vi "Parse Response Message.vi"(8 "error in":errorcluster, 11 "Luminos in":refnum<class "Luminos.lvclass">) -> (0 "error out":errorcluster, 3 "Luminos out":refnum<class "Luminos.lvclass">)   [LabVIEW 2018, in "Luminos.lvlib" / "Luminos.lvclass"]
uses:
  Luminos.lvclass
  Luminos.lvclass/Luminos.ctl
  PPLs/Axis/Axis.lvlibp/Axis.lvclass
  C:/Projects/LabVIEW/PPLs/Axis/Axis.lvlibp/Axis.lvclass
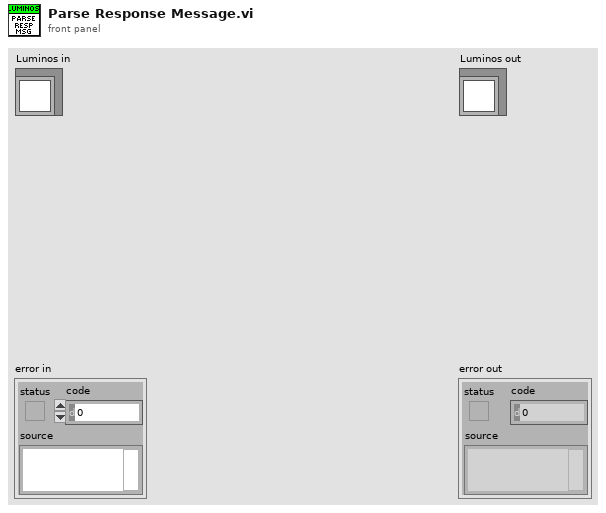
[diagram p1: front panel]
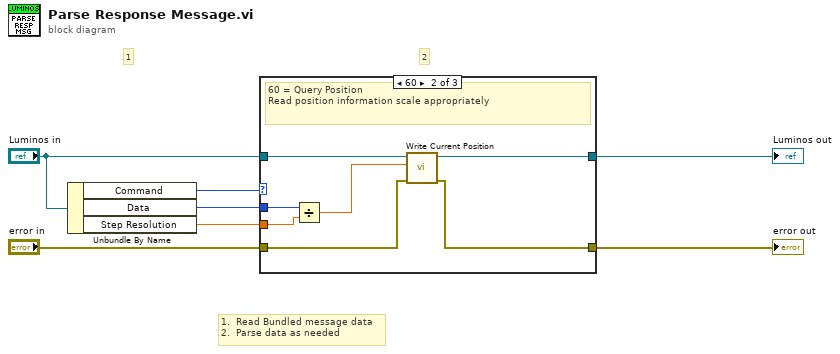
[diagram p0: block diagram]
diagram:
  # "2"
  # "1"
  # "1.  Read Bundled message data\n2.  Parse data as needed"
  n1 = Unbundle By Name("Luminos in") -> ("Command"=w5:u8, "Data"=w4:i32, "Step Resolution"=w1:dbl)
  n2 = case shown="60" w5 {
    tunnel: "Luminos in" -> [w9 w16 w18]
    tunnel: [w9 w15 w18] -> w6
    tunnel: w4 -> [_ w14 _]
    tunnel: "error in" -> [w8 w11 w17]
    tunnel: [w8 w10 w17] -> w2
    tunnel: w1 -> [_ w12 _]
    frame 0, Default {
      # "Any message that doesnt require parsing"
    }
    frame 60 {
      # "60 = Query Position \nRead position information scale appropriately"
      n3 = Divide(x=w14, y=w12) -> (x/y=w13:dbl)
      n4 = call "Write Current Position.vi"("error in"=w11, "Current Position"=w13, "Axis in"=w16) -> ("error out"=w10:errorcluster, "Axis out"=w15:refnum<class "Luminos.lvclass">)  [unwired: 7 in]
    }
    frame 54 {
      # "54 = Status - So far no status data is reported"
    }
  }
  "error out" <- w2
  "Luminos out" <- w6
